vi "OCR_Test_RH_24Jul21.vi"(5 "Image File Path":path=path "C:/images/img1.jpeg", 9 "Image in":T2(plugin-control), 12 "error in (no error)":errorcluster) -> (2 "OCR 3 Digit":T1, 3 "Read Center":string, 6 "Read Top":string caption="Read String", 10 "Image":T2(plugin-control), 14 "Read bottom":string, 15 "error out":errorcluster)   [LabVIEW 2019]
uses:
  <vilib>/vision/NI_Vision_Development_Module.lvlib
panel:
  in  "Training File Path":path=path "D:/Focusing Station/Sub VIs/OCR_Test_Right.abc"
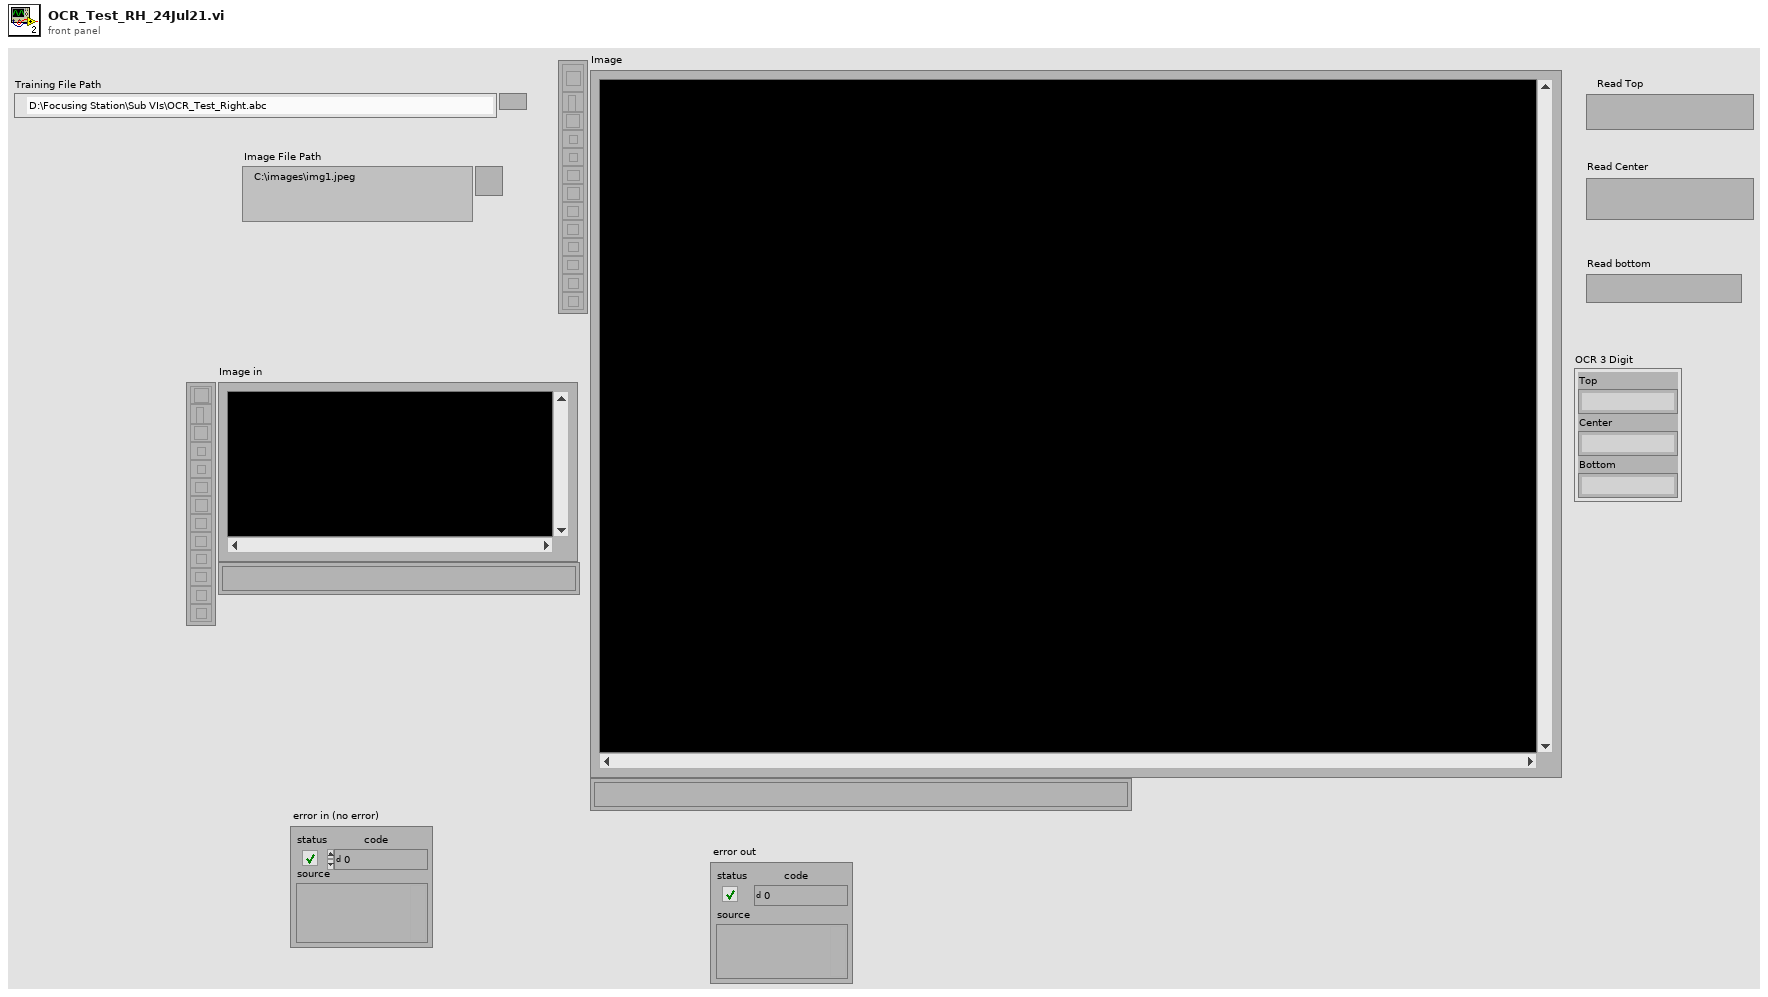
[diagram p1: front panel]
types:
  T1 = cluster{"Top":string, "Center":string, "Bottom":string}
  T2 = typedef "IMAQ Image.ctl" = refnum<image>
  T3 = typedef "IMAQ Rectangle" = cluster{"Left":i32, "Top":i32, "Right":i32, "Bottom":i32, "Rotation":dbl}
  T4 = typedef "Image Type" = u32
  T5 = typedef "IMAQ OCR Session.ctl" = refnum<k1>
  T6 = typedef "ROI Descriptor" = cluster{"Global Rectangle":i32[], "Contours":cluster{"ID":enum32{"External", "Internal"}, "Type":u32, "Coordinates":i32[]}[]}
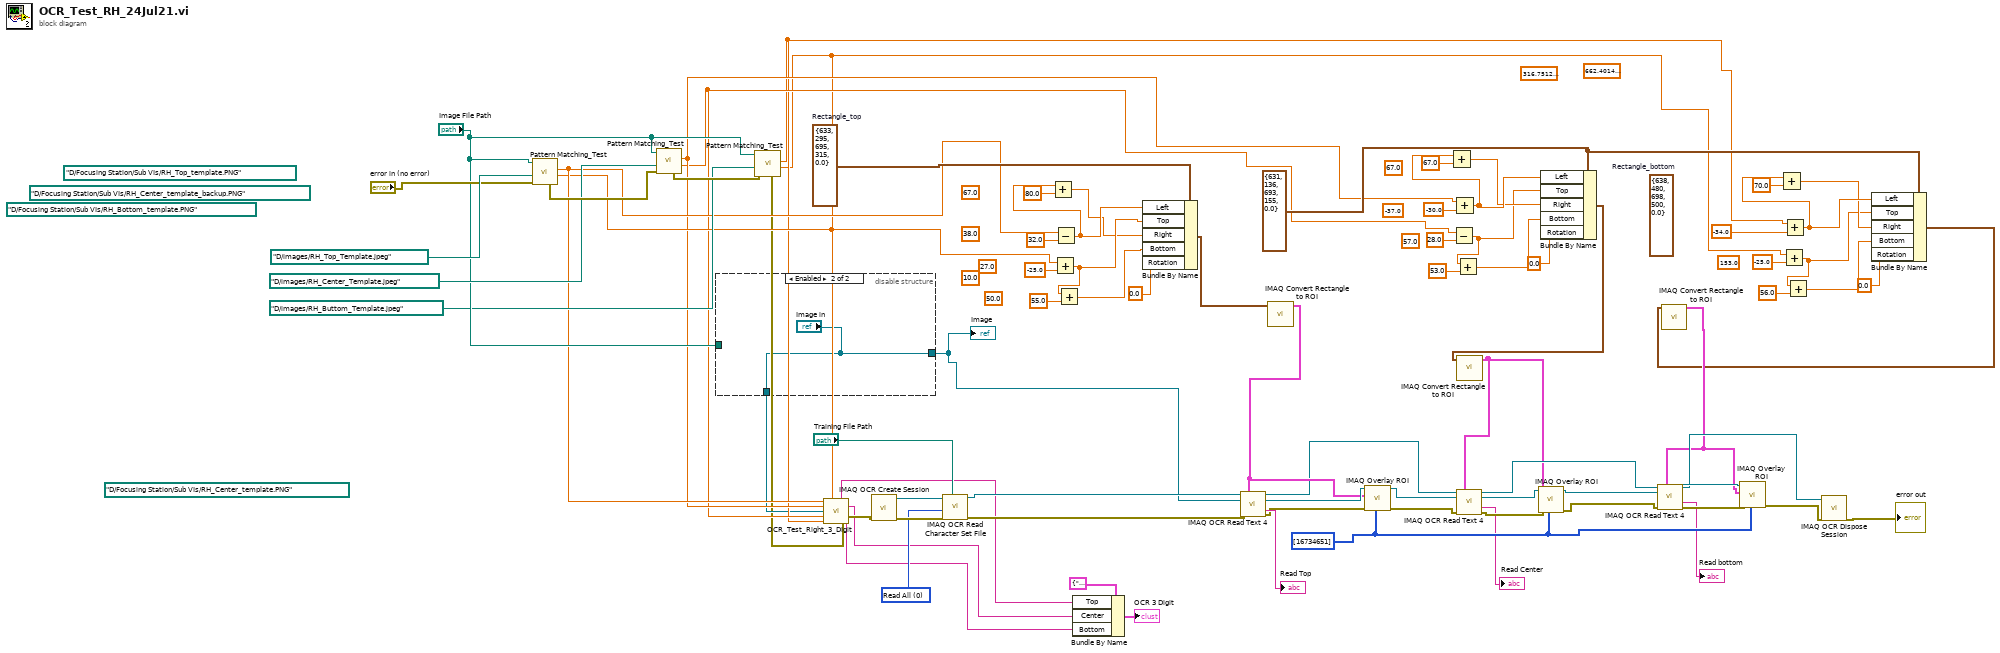
[diagram p0: block diagram]
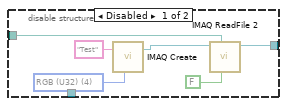
[diagram p2: hidden frame]
diagram:
  (unwired) sgl 67.0 ("y")
  (unwired) sgl -37.0 ("y")
  (unwired) sgl 10.0 ("y")
  (unwired) path "D:/Focusing Station/Sub VIs/RH_Bottom_template.PNG" ("Template file path")
  (unwired) path "D:/Focusing Station/Sub VIs/RH_Center_template_backup.PNG" ("Template file path")
  (unwired) path "D:/Focusing Station/Sub VIs/RH_Top_template.PNG" ("Template file path")
  (unwired) path "D:/Focusing Station/Sub VIs/RH_Center_template.PNG" ("Template file path")
  (unwired) sgl 50.0 ("y")
  (unwired) sgl 27.0 ("y")
  (unwired) sgl 67.0 ("y")
  (unwired) sgl 38.0 ("y")
  (unwired) sgl 153.0 ("y")
  (unwired) sgl 57.0 ("y")
  (unwired) sgl 316.75128 ("y")
  (unwired) sgl 662.4014 ("x")
  (unwired) T3 {"Left"=638, "Top"=480, "Right"=698, "Bottom"=500, "Rotation"=0.0}  # Rectangle_bottom
  w35 = T3 {"Left"=631, "Top"=136, "Right"=693, "Bottom"=155, "Rotation"=0.0}
  w73 = 0 items=["Read All", "Read Character Set Only", "Read Properties Only"] ("Read Options")
  w28 = T3 {"Left"=633, "Top"=295, "Right"=695, "Bottom"=315, "Rotation"=0.0}  # Rectangle_top
  w58 = u32[] [16734651] ("Colors (Green)")
  n1 = call "Pattern Matching_Test.vi"("error in (no error)"="error in (no error)", "Template file path"=path "D:/images/RH_Top_Template.jpeg", "File Path"="Image File Path") -> ("y"=w14:sgl, "x"=w15:sgl, "error out"=w20:errorcluster)  [unwired: 4 in, 2 out]
  n2 = call "Pattern Matching_Test.vi"("error in (no error)"=w20, "Template file path"=path "D:/images/RH_Center_Template.jpeg", "File Path"="Image File Path") -> ("y"=w12:sgl, "x"=w13:sgl, "error out"=w18:errorcluster)  [unwired: 4 in, 2 out]
  n3 = disable-structure shown="Enabled" {
    disable-tunnel: [w84 "Image in"] -> w77
    disable-tunnel: "Image File Path" -> [w83 _]
    disable-tunnel: [_ "Image in"] -> w9
    frame Disabled {
      w85 = T4 4 items=["Grayscale (U8)", "Grayscale (I16)", "Grayscale (SGL)", "Complex (CSG)", "RGB (U32)", "HSL (U32)", "RGB (U64)", "Grayscale (U16)"] ("Image Type")
      n4 = call "IMAQ Create"("Image Name"="Test", "Image Type"=w85) -> ("New Image"=w87:T2)  [unwired: 3 in, 1 out]
      n5 = call "IMAQ ReadFile 2"("Use File Path Image Type"=FALSE, "File Path"=w83, "Image"=w87) -> ("Image Out"=w84:T2)  [unwired: 4 in, 4 out]
    }
    frame Enabled {
    }
  }
  "Image" <- w77
  n6 = call "Pattern Matching_Test.vi"("error in (no error)"=w18, "Template file path"=path "D:/images/RH_Buttom_Template.jpeg", "File Path"="Image File Path") -> ("y"=w10:sgl, "x"=w11:sgl, "error out"=w7:errorcluster)  [unwired: 4 in, 2 out]
  n7 = call "OCR_Test_Right_3_Digit.vi"("x Top"=w15, "y Top"=w14, "x Center"=w13, "Image in"=w9, "y Center"=w12, "x Bottom"=w11, "y Bottom"=w10, "error in"=w7) -> ("Read Top"=w5:string, "Read Center"=w4:string, "error out"=w8:errorcluster, "Read bottom"=w6:string)  [unwired: 4 in]
  n8 = call "IMAQ OCR Create Session"("error in (no error)"=w8) -> ("error out"=w81:errorcluster, "IMAQ OCR Session"=w82:T5)  [unwired: 9 in]
  n9 = call "IMAQ OCR Read Character Set File"("File Path"="Training File Path", "error in (no error)"=w81, "Read Options"=w73, "IMAQ OCR Session"=w82) -> ("error out"=w78:errorcluster, "IMAQ OCR Session (dup)"=w79:T5)  [unwired: 5 in, 1 out]
  n10 = Add(x=w14, y=sgl -25.0) -> (x+y=w26:sgl)
  n11 = Subtract(x=w15, y=sgl 32.0) -> (x-y=w27:sgl)
  n12 = Add(x=w27, y=sgl 80.0) -> (x+y=w25:sgl)
  n13 = Add(x=w26, y=sgl 55.0) -> (x+y=w24:sgl)
  n14 = Bundle By Name(cluster=T1 {"Top"="", "Center"="", "Bottom"=""}, "Top"=w5, "Center"=w4, "Bottom"=w6) -> (→"OCR 3 Digit":T1)
  n15 = Bundle By Name(cluster=w28, "Left"=w27, "Top"=w26, "Right"=w25, "Bottom"=w24, "Rotation"=0.0) -> (w23:T3)
  n16 = call "IMAQ Convert Rectangle to ROI"("Rectangle"=w23) -> ("ROI Descriptor"=w72:T6)  [unwired: 8 in, 1 out]
  n17 = call "IMAQ OCR Read Text 4"("IMAQ OCR Session"=w79, "ROI Descriptor"=w72, "Image"=w77, "error in (no error)"=w78) -> ("IMAQ OCR Session (dup)"=w68:T5, "Image (dup)"=w74:T2, "Read String"=→"Read Top":string, "error out"=w75:errorcluster)  [unwired: 5 in, 3 out]
  n18 = call "IMAQ Overlay ROI"("Colors (Green)"=w58, "error in (no error)"=w75, "ROI Descriptor"=w72, "Image"=w74) -> ("error out"=w66:errorcluster, "Image Out"=w67:T2)  [unwired: 2 in, 4 out]
  n19 = Subtract(x=w12, y=sgl 28.0) -> (x-y=w46:sgl)
  n20 = Add(x=w13, y=sgl -30.0) -> (x+y=w48:sgl)
  n21 = Add(x=w48, y=sgl 67.0) -> (x+y=w47:sgl)
  n22 = Add(x=w46, y=sgl 53.0) -> (x+y=w45:sgl)
  n23 = Bundle By Name(cluster=w35, "Left"=w48, "Top"=w46, "Right"=w47, "Bottom"=w45, "Rotation"=0.0) -> (w44:T3)
  n24 = call "IMAQ Convert Rectangle to ROI"("Rectangle"=w44) -> ("ROI Descriptor"=w54:T6)  [unwired: 8 in, 1 out]
  n25 = call "IMAQ OCR Read Text 4"("IMAQ OCR Session"=w68, "ROI Descriptor"=w54, "Image"=w67, "error in (no error)"=w66) -> ("IMAQ OCR Session (dup)"=w61:T5, "Image (dup)"=w70:T2, "Read String"=→"Read Center":string, "error out"=w69:errorcluster)  [unwired: 5 in, 3 out]
  n26 = call "IMAQ Overlay ROI"("Colors (Green)"=w58, "error in (no error)"=w69, "ROI Descriptor"=w54, "Image"=w70) -> ("error out"=w62:errorcluster, "Image Out"=w63:T2)  [unwired: 2 in, 4 out]
  n27 = Add(x=w10, y=sgl -25.0) -> (x+y=w37:sgl)
  n28 = Add(x=w11, y=sgl -34.0) -> (x+y=w39:sgl)
  n29 = Add(x=w39, y=sgl 70.0) -> (x+y=w38:sgl)
  n30 = Add(x=w37, y=sgl 56.0) -> (x+y=w36:sgl)
  n31 = Bundle By Name(cluster=w35, "Left"=w39, "Top"=w37, "Right"=w38, "Bottom"=w36, "Rotation"=0.0) -> (w34:T3)
  n32 = call "IMAQ Convert Rectangle to ROI"("Rectangle"=w34) -> ("ROI Descriptor"=w57:T6)  [unwired: 8 in, 1 out]
  n33 = call "IMAQ OCR Read Text 4"("IMAQ OCR Session"=w61, "ROI Descriptor"=w57, "Image"=w63, "error in (no error)"=w62) -> ("IMAQ OCR Session (dup)"=w60:T5, "Image (dup)"=w64:T2, "Read String"=→"Read bottom":string, "error out"=w65:errorcluster)  [unwired: 5 in, 3 out]
  n34 = call "IMAQ Overlay ROI"("Colors (Green)"=w58, "error in (no error)"=w65, "ROI Descriptor"=w57, "Image"=w64) -> ("error out"=w59:errorcluster)  [unwired: 2 in, 5 out]
  n35 = call "IMAQ OCR Dispose Session"("error in (no error)"=w59, "IMAQ OCR Session"=w60) -> ("error out"=→"error out":errorcluster)  [unwired: 9 in]
